vi "niRFUtil WFM Replace Waveform Segment (complex wfm).vi"(4 "Waveform Segment":T2 {"y" format="%.2f"; "dx" format="%^.2e"; "x0" format="%^.2e"}, 5 "WFM replace mode":T1, 6 "Default Value (0)":sgl min=0 max=127 format="%.2f", 7 "Waveform In":T2 {"y" format="%.2f"; "dx" format="%^.2e"; "x0" format="%^.2e"}) -> (3 "Waveform Out":T2 {"y" format="%.2f"; "dx" format="%^.2e"; "x0" format="%^.2e"})   [LabVIEW 2015, in "niRFUtil.lvlib"]
doc: "(c) Copyright 2006, National Instruments, Inc. This VI may not be duplicated, sold, or distributed without written consent from National Instruments."
uses:
  niRFUtil.lvlib
  Includes/niRFUtil INC Complex Waveform.ctl
  Includes/niRFUtil INC Complex Array.ctl
  Includes/niRFUtil INC Waveform Replace Mode.ctl
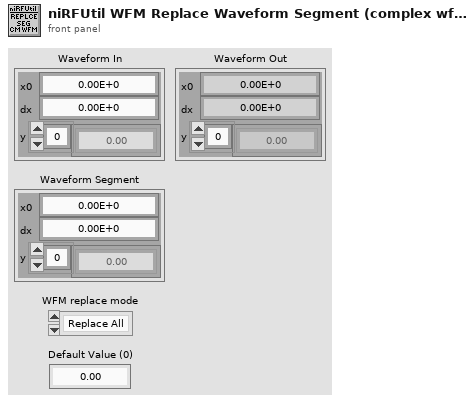
[diagram p1: front panel]
types:
  T1 = typedef "niRFUtil.lvlib/niRFUtil INC Waveform Replace Mode.ctl" = enum16{"Replace All", "Replace Pt By Pt"}
  T2 = typedef "niRFUtil.lvlib/niRFUtil INC Complex Waveform.ctl" = cluster{"x0":dbl, "dx":dbl, "y":T3}
  T3 = typedef "niRFUtil.lvlib/niRFUtil INC Complex Array.ctl" = csg[]
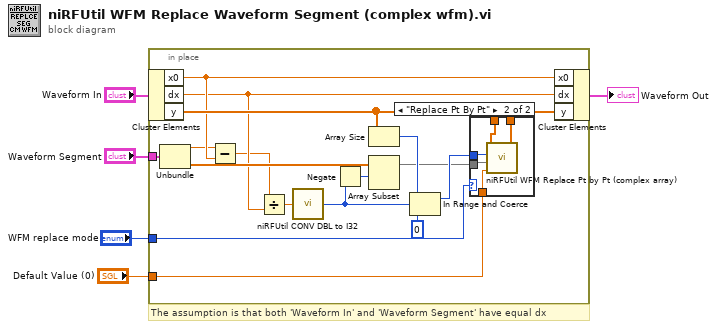
[diagram p0: block diagram]
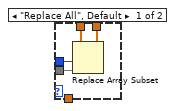
[diagram p2: hidden frame]
diagram:
  # "The assumption is that both 'Waveform In' and 'Waveform Segment' have equal dx"
  n1 = in-place {
    in-place-border: "Waveform Segment" -> [w19]
    in-place-border: "WFM replace mode" -> [w13]
    in-place-border: "Default Value (0)" -> [w12]
    n2 = in-place-cluster #1("Waveform In") -> ("x0"=w11:dbl, "dx"=w9:dbl, "y"=w15:T3)
    n3 = Unbundle(w19) -> ("x0"=w10:dbl, "y"=w17:T3)  [unwired: 1 out]
    n4 = Subtract(x=w10, y=w11) -> (x-y=w8:dbl)
    n5 = Divide(x=w8, y=w9) -> (x/y=w7:dbl)
    n6 = call "niRFUtil CONV DBL to I32.vi"("Numeric (DBL)"=w7) -> ("Numeric (I32)"=w6:i32)  [unwired: 14 in]
    n7 = Negate(x=w6) -> (-x=w18:i32)
    n8 = Array Size(array=w15) -> (size(s)=w21:i32)
    n9 = Array Subset(array=w17, index=w18) -> (w16:T3)  [unwired: 1 in]
    n10 = In Range and Coerce(upper limit=w21, x=w6, lower limit=0) -> (coerced(x)=w20:i32)  [unwired: 1 out]
    n11 = case shown="\"Replace Pt By Pt\"" w13 {
      tunnel: w20 -> [w26 w29]
      tunnel: w16 -> [w25 w28]
      tunnel: w15 -> [w24 w31]
      tunnel: [w23 w30] -> w14
      tunnel: w12 -> [_ w27]
      frame "Replace All", Default {
        n12 = Replace Array Subset(array=w24, new element=w25, index=w26) -> (w23:T3)
      }
      frame "Replace Pt By Pt" {
        n13 = call "niRFUtil WFM Replace Pt by Pt (complex array).vi"("Complex Array In"=w31, "Replace Index"=w29, "Replace With"=w28, "Default Value (0)"=w27) -> ("Complex Array Out"=w30:T3)  [unwired: 2 in]
      }
    }
    n14 = in-place-cluster #1("x0"=w11, "dx"=w9, "y"=w14) -> (→"Waveform Out":T2)
  }
